vi "Excel - Write Table.vi"() -> ()   [LabVIEW 2023]
doc: "This VI demonstrates the use of ActiveX to write a table into a Microsoft Excel worksheet."
panel:
  in  "Table":string[][](table)=[["1", "2", "3", "4", "5", "6", "7", "8", "9", "10"], ["10", "11", "12", "13", "14", "15", "16", "17", "18", "19"], ["20", "21", "22", "23", "24", "25", "26", "27", "28", "29"], ["30", "31", "32", "33", "34", "35", "36", "37", "38", "39"]]
  # "Overview: Demonstrates how to write table data to an Excel worksheet.\nRequirements: Windows with Microsoft Excel\nInstructions:\nRun the VI."
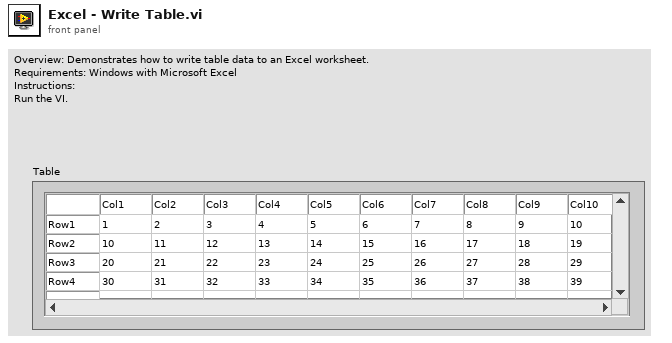
[diagram p1: front panel]
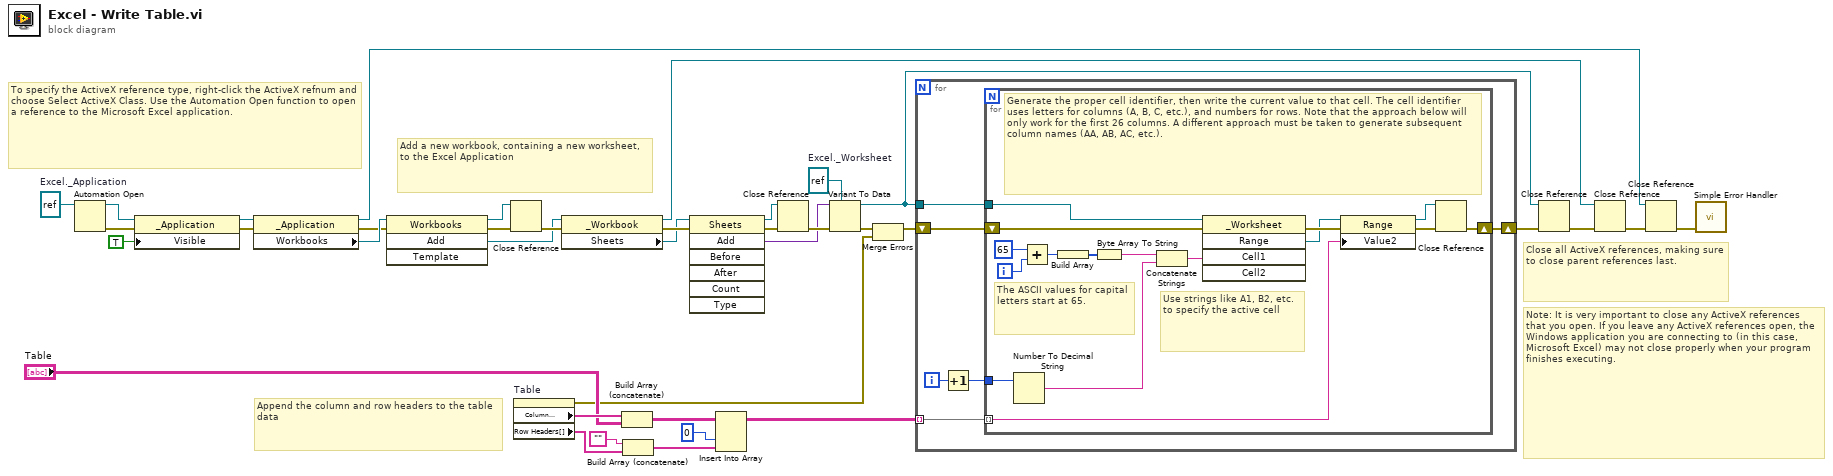
[diagram p0: block diagram]
diagram:
  w15 = refnum<k7> refnum  # Excel._Worksheet
  w31 = refnum<k7> refnum  # Excel._Application
  # "Note: It is very important to close any ActiveX references that you open. If you leave any ActiveX references open, the Windows application you are connecting to (in this case, Microsoft Excel) may not close properly when your program finishes executing."
  # "Add a new workbook, containing a new worksheet, to the Excel Application"
  # "Append the column and row headers to the table data"
  # "Close all ActiveX references, making sure to close parent references last."
  # "To specify the ActiveX reference type, right-click the ActiveX refnum and choose Select ActiveX Class. Use the Automation Open function to open a reference to the Microsoft Excel application."
  n1 = Automation Open(Automation Refnum=w31) -> (Automation Refnum=w32:refnum<k7>, error out=w33:errorcluster)  [unwired: 1 in, 2 out]
  n2 = property class="_Application"(reference=w32, error in=w33, "Visible"=TRUE) -> (reference out=w24:refnum<k7>, error out=w26:errorcluster)
  n3 = property class="_Application"(reference=w24, error in=w26) -> (reference out=w21:refnum<k7>, error out=w29:errorcluster, "Workbooks"=w30:refnum<k7>)
  n4 = invoke class="Workbooks" method="Add"(reference=w30, error in=w29) -> (reference out=w27:refnum<k7>, error out=w28:errorcluster, "Add"=w22:refnum<k7>)  [unwired: 2 in, 1 out]
  n5 = Close Reference(reference=w27, error in (no error)=w28) -> (error out=w23:errorcluster)
  n6 = property on="Table" class="Tbl (strict)"() -> (error out=w4:errorcluster, "Column Headers[]"=w10:string[], "Row Headers[]"=w3:string[])  [unwired: 2 in, 1 out]
  n7 = property class="_Workbook"(reference=w22, error in=w23) -> (reference out=w19:refnum<k7>, error out=w13:errorcluster, "Sheets"=w12:refnum<k7>)
  n8 = Build Array (concatenate)(w10, "Table") -> (w8:string[][])
  n9 = Build Array (concatenate)("", w3) -> (w2:string[])
  n10 = invoke class="Sheets" method="Add"(reference=w12, error in=w13) -> (reference out=w16:refnum<k7>, error out=w17:errorcluster, "Add"=w14:variant)  [unwired: 5 in, 4 out]
  n11 = Insert Into Array(array=w8, index (col)=0 ("disabled index (col)"), new element=w2) -> (w6:string[][])  [unwired: 1 in]
  n12 = Close Reference(reference=w16, error in (no error)=w17) -> (error out=w18:errorcluster)
  n13 = Variant To Data(error in=w18, type=w15, Variant=w14) -> (data=w20:refnum<k7>, error out=w11:errorcluster)
  n14 = Merge Errors(w11, w4) -> (w5:errorcluster)
  n15 = for {
    shift-right: [w42] -> w34
    shift-left: w5 -> [w43]
    tunnel: w20 -> [w41]
    tunnel: w6 -> [w38] mode=indexing
    i -> [w40]
    n16 = Increment(x=w40) -> (x+1=w39:i32)
    n17 = for {
      shift-right: [w55] -> w42
      shift-left: w43 -> [w53]
      tunnel: w41 -> [w52]
      tunnel: w39 -> [w47]
      tunnel: w38 -> [w57] mode=indexing
      i -> [w48]
      # "Use strings like A1, B2, etc. to specify the active cell"
      # "The ASCII values for capital letters start at 65."
      # "Generate the proper cell identifier, then write the current value to that cell. The cell identifier uses letters for columns (A, B, C, etc.), and numbers for rows. Note that the approach below will only work for the first 26 columns. A different approach must be taken to generate subsequent column names (AA, AB, AC, etc.)."
      n18 = Number To Decimal String(number=w47) -> (decimal integer string=w45:string)  [unwired: 1 in]
      n19 = Add(x=65, y=w48) -> (x+y=w50:i32)
      n20 = Build Array(w50) -> (w49:i32[])
      n21 = Byte Array To String(unsigned byte array=w49) -> (string=w46:string)
      n22 = Concatenate Strings(w46, w45) -> (w44:string)
      n23 = invoke class="_Worksheet" method="Range"(reference=w52, error in=w53, "Cell1"=w44) -> (error out=w59:errorcluster, "Range"=w58:refnum<k7>)  [unwired: 2 in, 3 out]
      n24 = property class="Range"(reference=w58, error in=w59, "Value2"=w57) -> (reference out=w54:refnum<k7>, error out=w56:errorcluster)
      n25 = Close Reference(reference=w54, error in (no error)=w56) -> (error out=w55:errorcluster)
    }
  }
  n26 = Close Reference(reference=w20, error in (no error)=w34) -> (error out=w37:errorcluster)
  n27 = Close Reference(reference=w19, error in (no error)=w37) -> (error out=w36:errorcluster)
  n28 = Close Reference(reference=w21, error in (no error)=w36) -> (error out=w35:errorcluster)
  n29 = call <vilib>:"Simple Error Handler.vi"("error in (no error)"=w35) -> ()  [unwired: 4 in, 5 out]
